vi "ScriptParser.vi"(0 "File Path Control":path, 1 "storage refnum (file) out":refnum<k20>, 2 "ResultaFileName":string, 3 "Array":string[](array[string]), 4 "I":dbl) -> ()   [LabVIEW 2014]
uses:
  <vilib>/Platform/storage/Storage.llb/usiSequenceRepresentation.ctl
  <vilib>/Platform/storage/lvStorage.llb/_queryPropPoly.vi
  <vilib>/Platform/storage/lvStorage.llb/_queryPropString.vi
  <vilib>/Platform/storage/lvStorage.llb/_queryGenericObjects.vi
  <vilib>/Platform/storage/lvStorage.llb/_loadAllDdt.vi
  <vilib>/Platform/storage/lvStorage.llb/xStorage/xStorageSupp/ErrorOut.vi
  <vilib>/Platform/storage/lvStorage.llb/_createOrGetByNameExplicitChildObject.vi
  <vilib>/Platform/storage/Storage.llb/__savePropString.vi
  <vilib>/Platform/storage/lvStorage.llb/__saveFloat64Channel.vi
  <vilib>/Platform/storage/lvStorage.llb/_openStorageWithRootAutoDetect.vi
  <vilib>/Platform/storage/Storage.llb/__savePropTime.vi
  <vilib>/Platform/storage/lvStorage.llb/xStorage/Read Data/Read Data.xnode
  <vilib>/Platform/storage/lvStorage.llb/xStorage/Write Data/Write Data.xnode
  <vilib>/Platform/storage/lvStorage.llb/xStorage/Open Data Storage/Open Data Storage.xnode
  <vilib>/Platform/storage/lvStorage.llb/xStorage/Set Properties/Set Properties.xnode
panel:
  out "Numeric":dbl
  out "storage refnums (channel)":refnum<k20>[](array[refnum])
  out "Default":bool
  # "DEBUG"
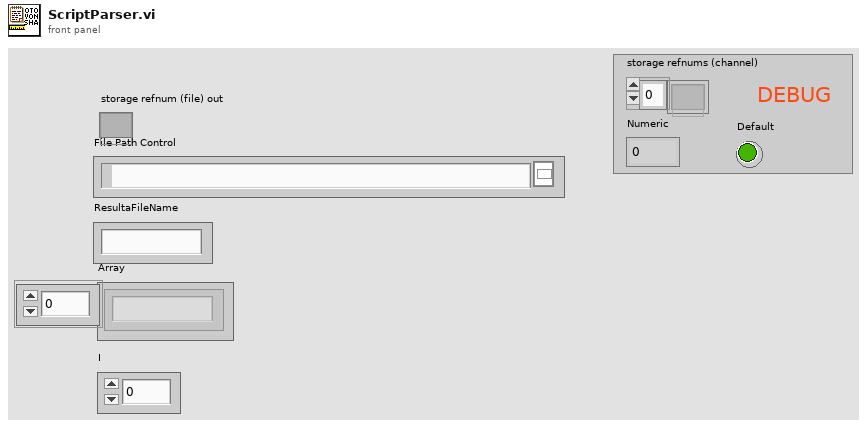
[diagram p1: front panel]
types:
  T1 = enum16{"UPDATE", "READ", "QUERY", "CREATE CHILD", "CREATE", "CONNECT", "DISCONNECT"}
  T2 = enum16{"Append values", "Replace values at index", "Replace all values"}
  T3 = typedef "usiSequenceRepresentation.ctl" = enum16{"explicit", "implicit"}
  T4 = enum16{"open", "open or create", "create or replace", "create", "open (read only)"}
  T5 = typedef "VBreakInitialCond.ctl" = cluster{"Range":dbl, "Ilim":dbl, "Level":dbl, "Channel":i32, "Timed Totalize":dbl}
  T6 = typedef "VBreakStopCondition.ctl" = cluster{"Count Min":dbl, "Count Max":dbl, "Vmax":dbl}
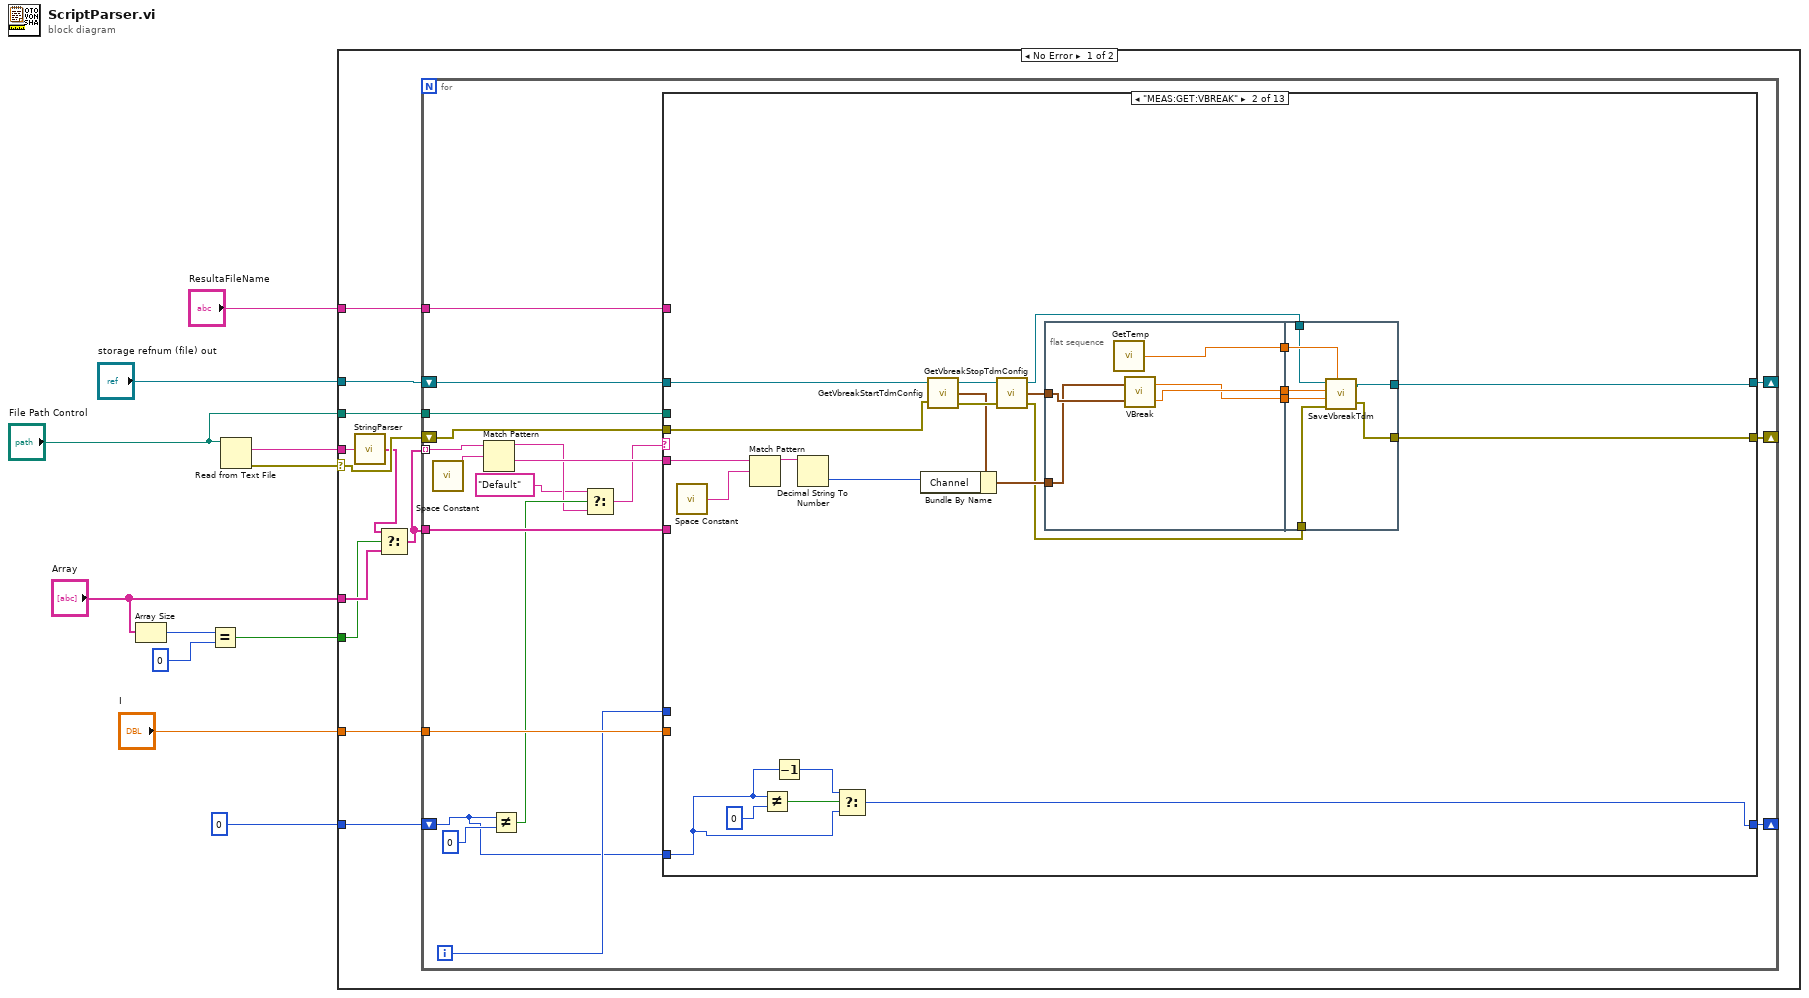
[diagram p0: block diagram]
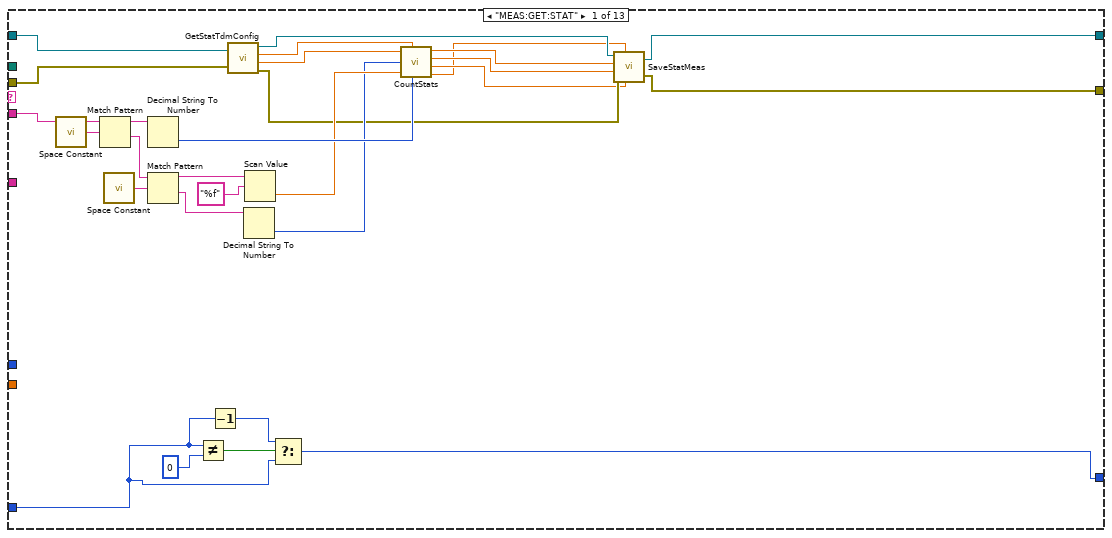
[diagram p2: hidden frame]
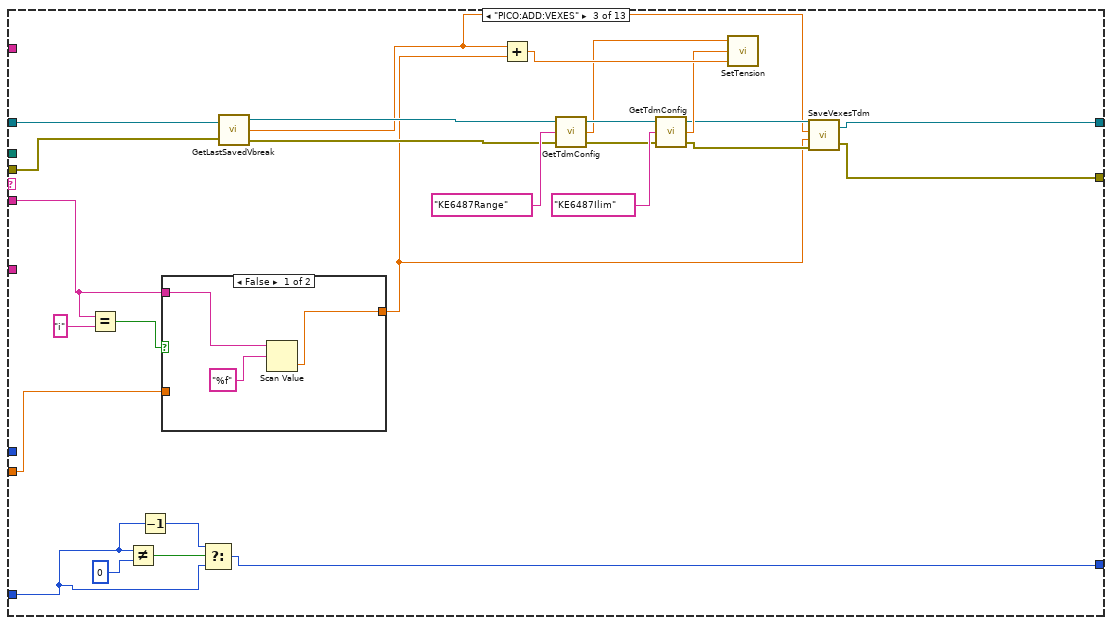
[diagram p3: hidden frame]
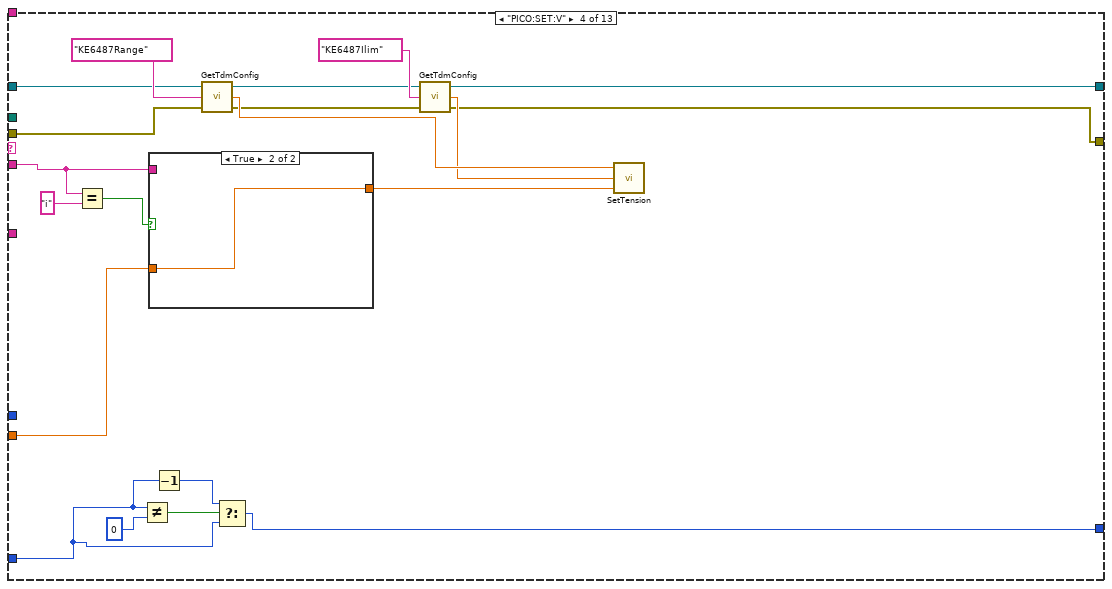
[diagram p5: hidden frame]
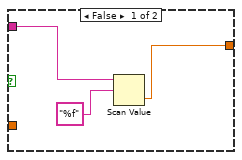
[diagram p6: hidden frame]
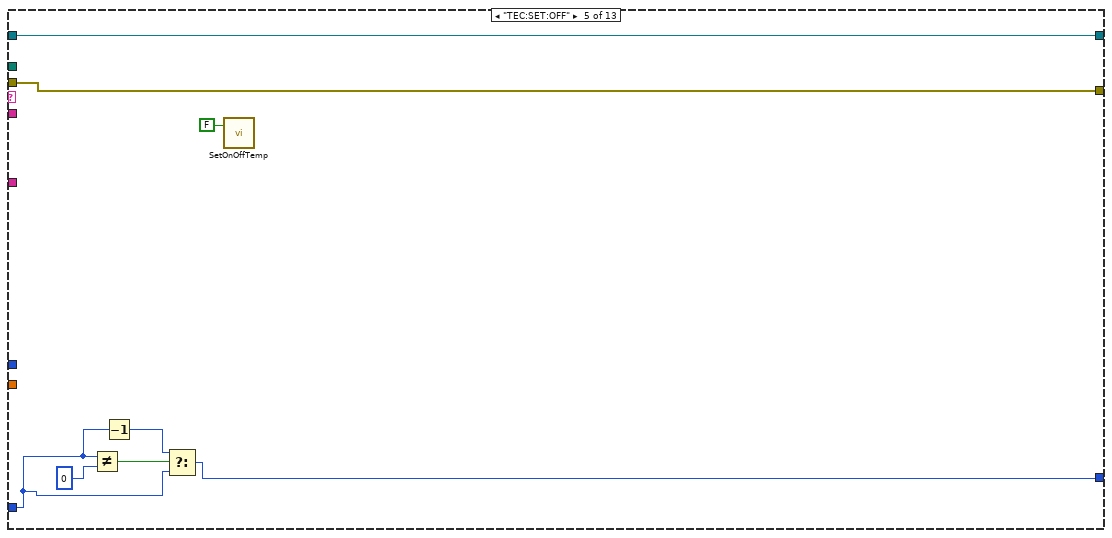
[diagram p7: hidden frame]
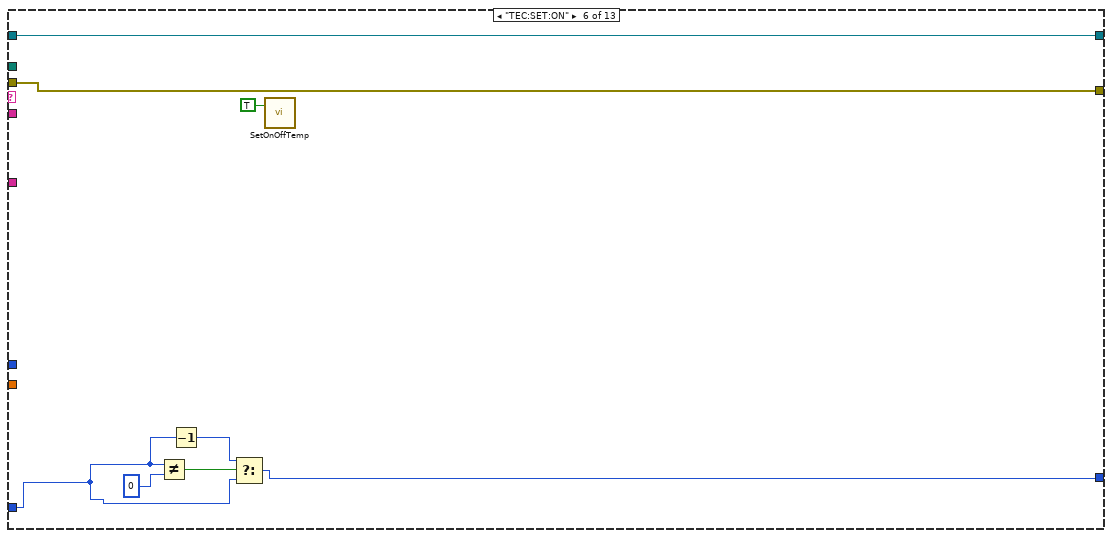
[diagram p8: hidden frame]
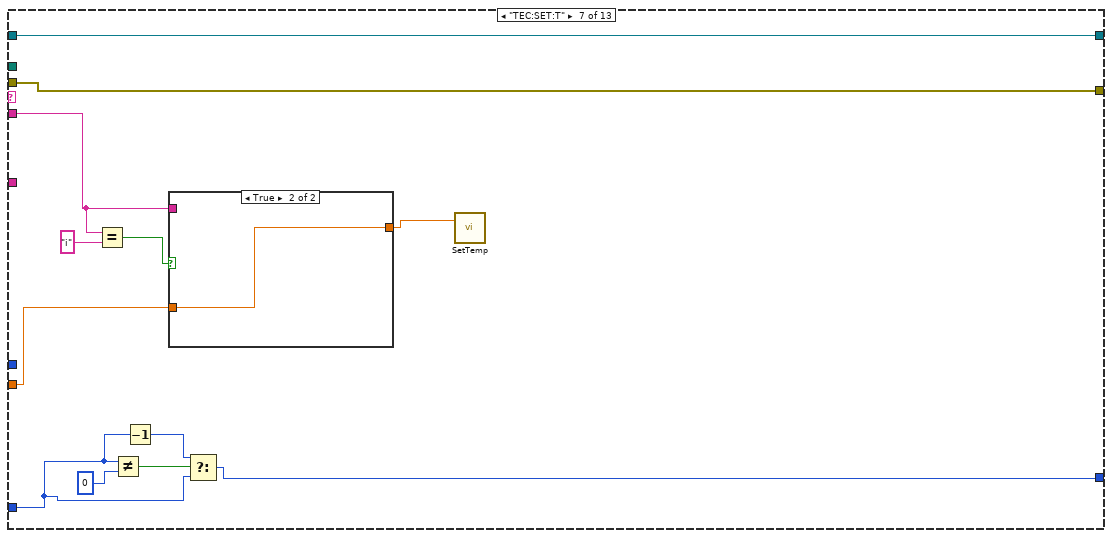
[diagram p9: hidden frame]
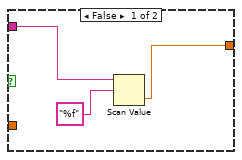
[diagram p10: hidden frame]
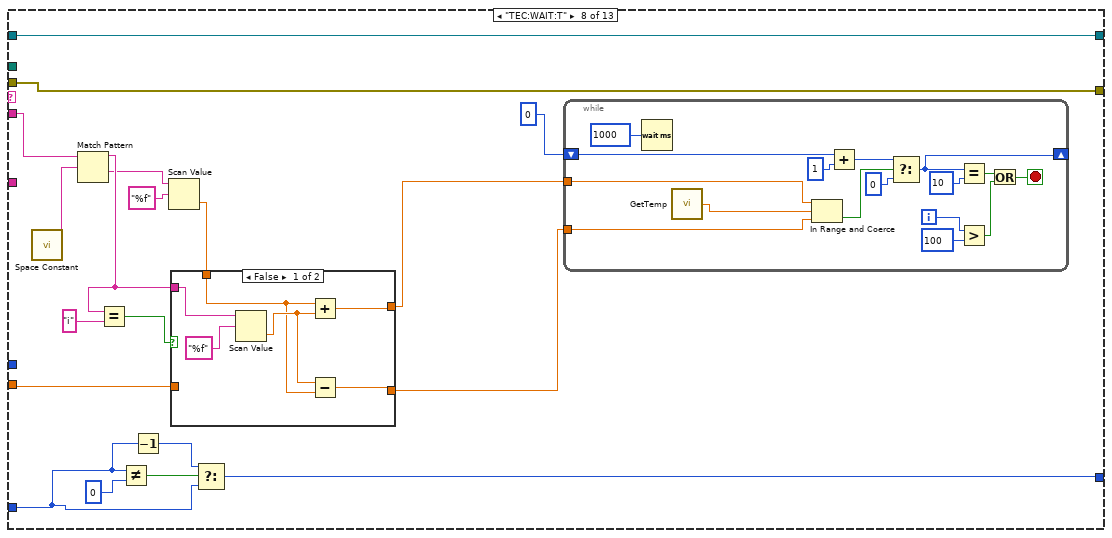
[diagram p11: hidden frame]
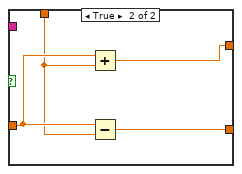
[diagram p12: hidden frame]
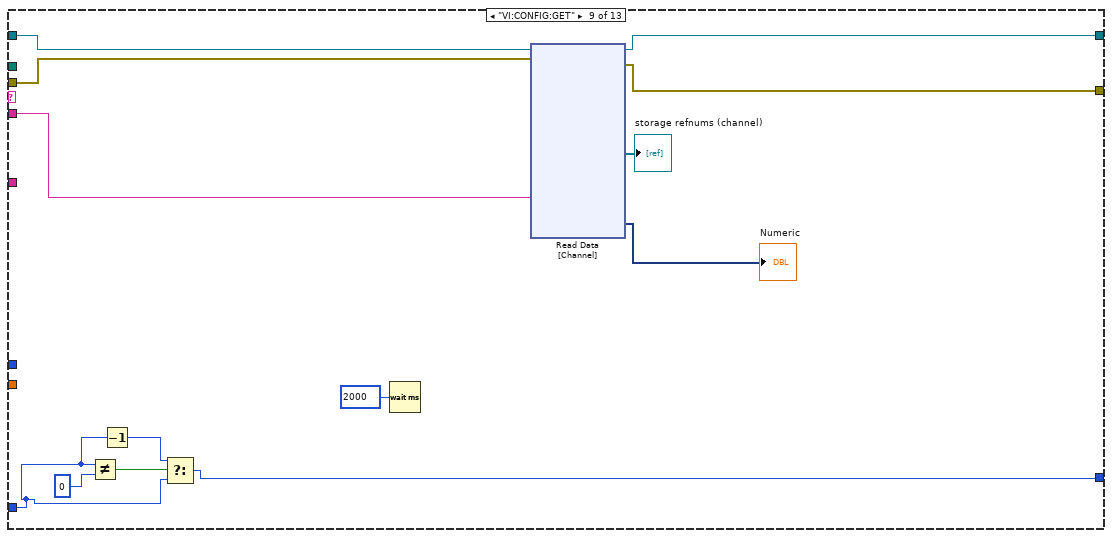
[diagram p13: hidden frame]
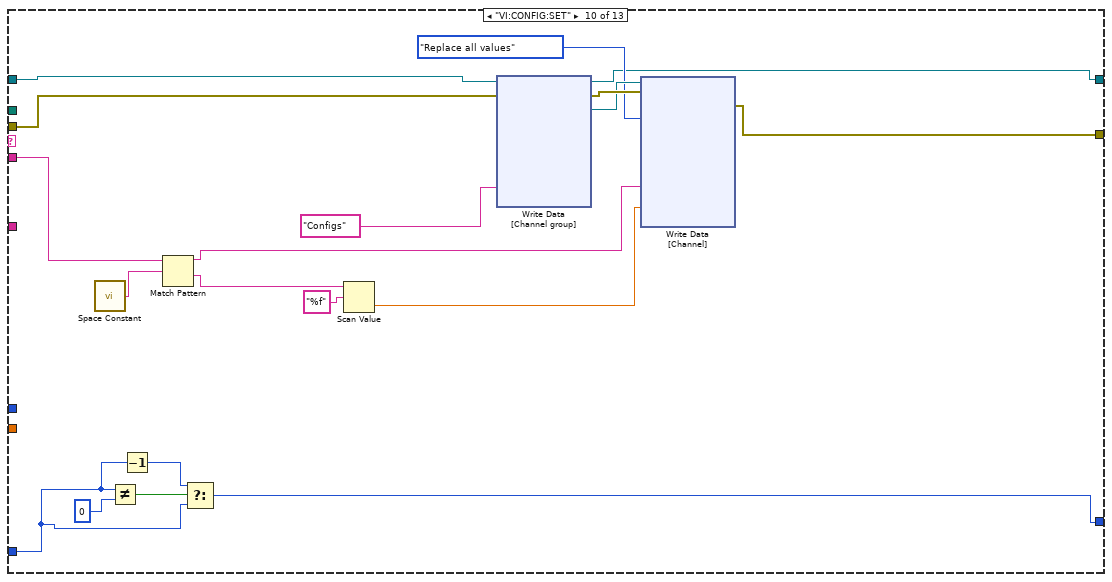
[diagram p14: hidden frame]
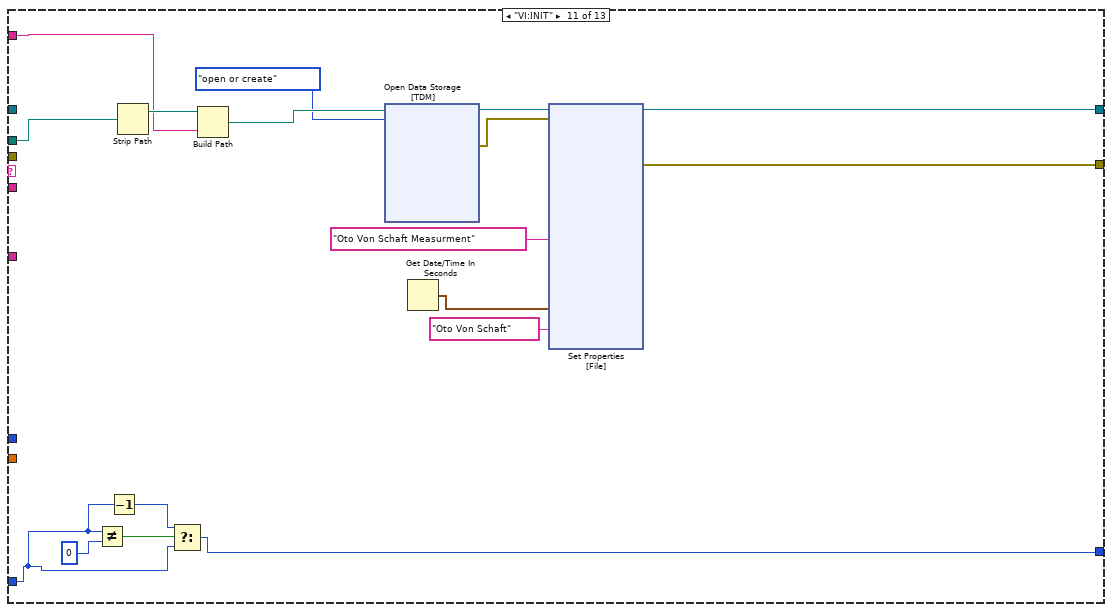
[diagram p15: hidden frame]
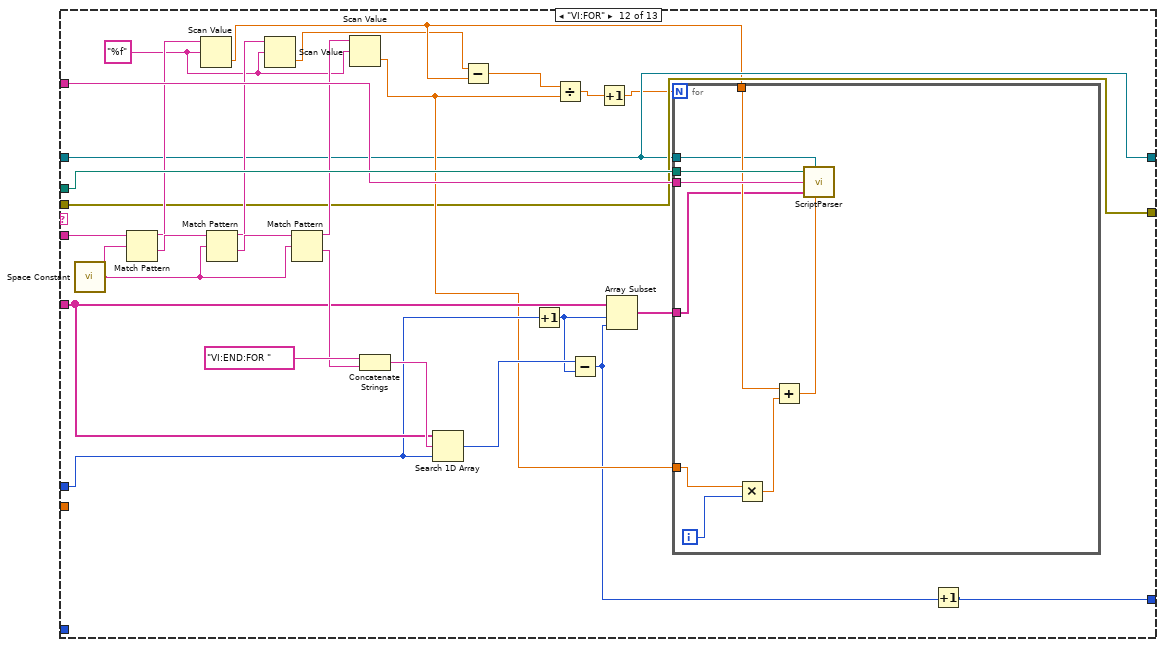
[diagram p16: hidden frame]
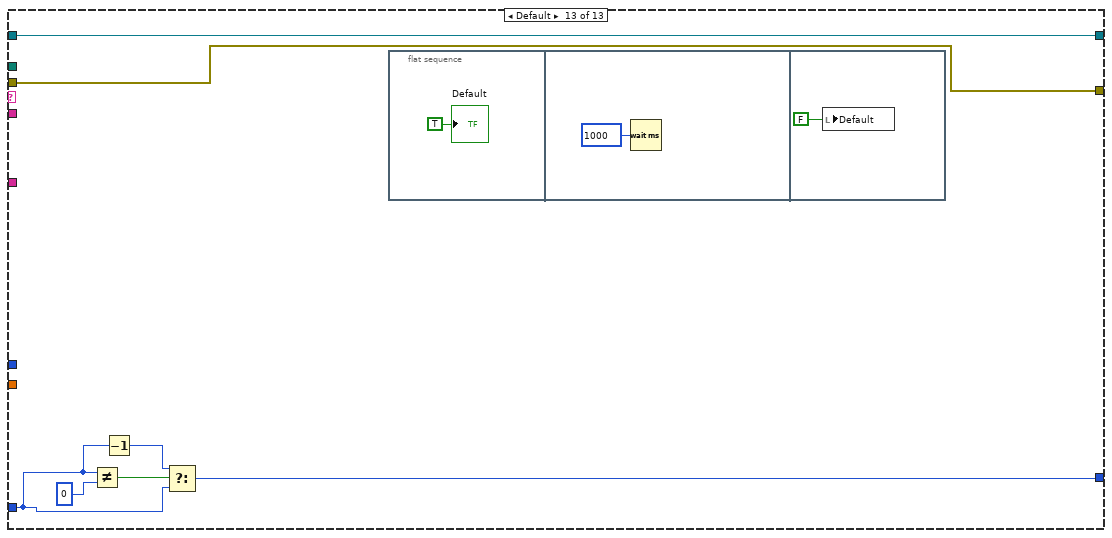
[diagram p17: hidden frame]
diagram:
  n1 = Array Size(array="Array") -> (size(s)=w4:i32)
  n2 = Equal?(x=w4, y=0) -> (x = y?=w2:bool)
  n3 = Read from Text File(file (use dialog)="File Path Control") -> (text=w6:string, error out=w11:errorcluster)  [unwired: 3 in, 2 out]
  n4 = case shown="No Error" w11 {
    selector: w11 -> [w20 _]
    tunnel: w6 -> [w18 _]
    tunnel: "File Path Control" -> [w22 _]
    tunnel: "ResultaFileName" -> [w21 _]
    tunnel: "I" -> [w19 _]
    tunnel: "storage refnum (file) out" -> [w17 _]
    tunnel: "Array" -> [w15 _]
    tunnel: w2 -> [w14 _]
    tunnel: 0 -> [w12 _]
    frame No Error {
      n5 = call "StringParser.vi"("String"=w18) -> ("array"=w16:string[])
      n6 = Select(t=w16, s=w14, f=w15) -> (s? t:f=w13:string[])
      n7 = for {
        tunnel: w13 -> [w40] mode=indexing
        tunnel: w22 -> [w35]
        tunnel: w21 -> [w38]
        shift-right: [w37] -> _
        shift-left: w17 -> [w34]
        shift-right: [w36] -> _
        shift-left: w20 -> [w33]
        tunnel: w19 -> [w32]
        tunnel: w13 -> [w31]
        shift-right: [w24] -> _
        shift-left: w12 -> [w23]
        i -> [w30]
        n8 = call <vilib>:"Space Constant.vi"() -> ("String"=w41:string)
        n9 = Match Pattern(string=w40, regular expression=w41) -> (before substring=w27:string, after substring=w39:string)  [unwired: 1 in, 2 out]
        n10 = Not Equal?(x=w23, y=0) -> (x != y?=w28:bool)
        n11 = Select(t="Default", s=w28, f=w27) -> (s? t:f=w25:string)
        n12 = case shown="\"MEAS:GET:VBREAK\"" w25 {
          tunnel: w39 -> [w66 w86 w112 w142 _ _ w181 w197 w248 w285 _ w397 _]
          tunnel: w35 -> [_ _ _ _ _ _ _ _ _ _ w333 w386 _]
          tunnel: w38 -> [_ _ _ _ _ _ _ _ _ _ w334 w384 _]
          tunnel: [w48 w71 w108 w146 w165 w173 w186 w207 w243 w274 w325 w376 w413] -> w37
          tunnel: [w47 w70 w107 w145 w164 w172 w185 w206 w242 w273 w324 w377 w412] -> w36
          tunnel: w34 -> [w69 w92 w130 w150 w165 w173 w186 w207 w244 w275 _ w376 w413]
          tunnel: w33 -> [w68 w91 w129 w149 w164 w172 w185 w206 w241 w272 _ w377 w412]
          tunnel: w32 -> [_ _ w111 w140 _ _ w182 w198 _ _ _ _ _]
          tunnel: w31 -> [_ _ _ _ _ _ _ _ _ _ _ w390 _]
          tunnel: w30 -> [_ _ _ _ _ _ _ _ _ _ _ w388 _]
          tunnel: [w42 w77 w117 w135 w159 w167 w175 w201 w236 w267 w319 w372 w407] -> w24
          tunnel: w23 -> [w43 w78 w118 w136 w160 w168 w176 w202 w237 w268 w320 _ w408]
          frame "MEAS:GET:STAT" {
            n13 = call <vilib>:"Space Constant.vi"() -> ("String"=w67:string)
            n14 = Match Pattern(string=w66, regular expression=w67) -> (before substring=w63:string, after substring=w60:string)  [unwired: 1 in, 2 out]
            n15 = call <vilib>:"Space Constant.vi"() -> ("String"=w61:string)
            n16 = Decimal String To Number(string=w63) -> (number=w62:i32)  [unwired: 2 in, 1 out]
            n17 = Match Pattern(string=w60, regular expression=w61) -> (before substring=w59:string, after substring=w57:string)  [unwired: 1 in, 2 out]
            n18 = Not Equal?(x=w43, y=0) -> (x != y?=w45:bool)
            n19 = Decrement(x=w43) -> (x-1=w44:i32)
            n20 = call "GetStatTdmConfig.vi"("storage refnum (file)"=w69, "error in"=w68) -> ("storage refnum (file) out"=w54:refnum<k20>, "Impedance"=w65:dbl, "Voltage Range"=w64:dbl, "error out"=w53:errorcluster)
            n21 = Decimal String To Number(string=w57) -> (number=w55:i32)  [unwired: 2 in, 1 out]
            n22 = Scan Value(string=w59, format string="%f") -> (value=w56:dbl)  [unwired: 1 in, 1 out]
            n23 = Select(t=w44, s=w45, f=w43) -> (s? t:f=w42:i32)
            n24 = call "CountStats.vi"("Voltage Range (5V)"=w64, "Impedance (1E+6 Ohm)"=w65, "Channel (Channel1)"=w55, "Totalize Timed (s)"=w56, "Points"=w62) -> ("Moyenne"=w52:dbl, "Ecart type"=w51:dbl, "Min"=w50:dbl, "Max"=w49:dbl)
            n25 = call "SaveStatMeas.vi"("Min"=w50, "Max"=w49, "error in"=w53, "Ecart Type"=w51, "Moyenne"=w52, "storage refnum (file)"=w54) -> ("error out"=w47:errorcluster, "storage refnum (file) 2"=w48:refnum<k20>)
          }
          frame "MEAS:GET:VBREAK" {
            n26 = call <vilib>:"Space Constant.vi"() -> ("String"=w87:string)
            n27 = Match Pattern(string=w86, regular expression=w87) -> (before substring=w85:string)  [unwired: 1 in, 3 out]
            n28 = Not Equal?(x=w78, y=0) -> (x != y?=w80:bool)
            n29 = Decrement(x=w78) -> (x-1=w79:i32)
            n30 = Decimal String To Number(string=w85) -> (number=w83:i32)  [unwired: 2 in, 1 out]
            n31 = Select(t=w79, s=w80, f=w78) -> (s? t:f=w77:i32)
            n32 = call "GetVbreakStartTdmConfig.vi"("storage refnum (file)"=w92, "error in"=w91) -> ("storage refnum (file) out"=w90:refnum<k20>, "output cluster"=w84:T5, "error out"=w89:errorcluster)
            n33 = Bundle By Name(cluster=w84, "Channel"=w83) -> (w82:T5)
            n34 = call "GetVbreakStopTdmConfig.vi"("storage refnum (file)"=w90, "error in"=w89) -> ("storage refnum (file) out"=w73:refnum<k20>, "output cluster"=w88:T6, "error out"=w72:errorcluster)
            n35 = flat-sequence {
              tunnel: w88 -> [w97]
              tunnel: w82 -> [w93]
              tunnel: [w96] -> w76
              tunnel: [w95] -> w75
              tunnel: [w94] -> w74
              tunnel: w76 -> [w103]
              tunnel: w75 -> [w102]
              tunnel: w74 -> [w104]
              tunnel: w73 -> [w100]
              tunnel: w72 -> [w101]
              tunnel: [w99] -> w71
              tunnel: [w98] -> w70
              frame #0 {
                n36 = call "GetTemp.vi"() -> ("result"=w94:dbl)
                n37 = call "VBreak.vi"("Condition d'arret"=w97, "Condition Initial"=w93) -> ("VBreak"=w96:dbl, "Count"=w95:dbl)
              }
              frame #1 {
                n38 = call "SaveVbreakTdm.vi"("storage refnum (file)"=w100, "Vbreak"=w103, "Count"=w102, "error in"=w101, "Temp"=w104) -> ("storage refnum (file) 2"=w99:refnum<k20>, "error out"=w98:errorcluster)
              }
            }
          }
          frame "PICO:ADD:VEXES" {
            n39 = Equal?(x=w112, y="i") -> (x = y?=w113:bool)
            n40 = Not Equal?(x=w118, y=0) -> (x != y?=w120:bool)
            n41 = Decrement(x=w118) -> (x-1=w119:i32)
            n42 = case shown="False" w113 {
              tunnel: w112 -> [w132 _]
              tunnel: [w131 w134] -> w105
              tunnel: w111 -> [_ w134]
              frame False {
                n43 = Scan Value(string=w132, format string="%f") -> (value=w131:dbl)  [unwired: 1 in, 1 out]
              }
              frame True {
              }
            }
            n44 = Select(t=w119, s=w120, f=w118) -> (s? t:f=w117:i32)
            n45 = call "GetLastSavedVbreak.vi"("storage refnum (file)"=w130, "error in"=w129) -> ("storage refnum (file) out"=w116:refnum<k20>, "VBreak"=w106:dbl, "error out"=w115:errorcluster)
            n46 = Add(x=w106, y=w105) -> (x+y=w124:dbl)
            n47 = call "GetTdmConfig.vi"("error in 2"=w115, "String"="KE6487Range", "storage refnum (file)"=w116) -> ("error in"=w125:errorcluster, "Numeric"=w123:dbl, "storage refnum (file) out"=w126:refnum<k20>)
            n48 = call "GetTdmConfig.vi"("error in 2"=w125, "String"="KE6487Ilim", "storage refnum (file)"=w126) -> ("error in"=w109:errorcluster, "Numeric"=w122:dbl, "storage refnum (file) out"=w110:refnum<k20>)
            n49 = call "SetTension.vi"("level"=w124, "compliance limit"=w122, "range"=w123) -> ()
            n50 = call "SaveVexesTdm.vi"("error in"=w109, "VExes"=w105, "Vbreak"=w106, "storage refnum (file)"=w110) -> ("error out"=w107:errorcluster, "storage refnum (file) 3"=w108:refnum<k20>)
          }
          frame "PICO:SET:V" {
            n51 = Equal?(x=w142, y="i") -> (x = y?=w143:bool)
            n52 = Not Equal?(x=w136, y=0) -> (x != y?=w138:bool)
            n53 = case shown="True" w143 {
              tunnel: w142 -> [w156 _]
              tunnel: [w155 w158] -> w141
              tunnel: w140 -> [_ w158]
              frame False {
                n54 = Scan Value(string=w156, format string="%f") -> (value=w155:dbl)  [unwired: 1 in, 1 out]
              }
              frame True {
              }
            }
            n55 = Decrement(x=w136) -> (x-1=w137:i32)
            n56 = call "GetTdmConfig.vi"("error in 2"=w149, "String"="KE6487Range", "storage refnum (file)"=w150) -> ("error in"=w147:errorcluster, "Numeric"=w154:dbl, "storage refnum (file) out"=w148:refnum<k20>)
            n57 = Select(t=w137, s=w138, f=w136) -> (s? t:f=w135:i32)
            n58 = call "GetTdmConfig.vi"("error in 2"=w147, "String"="KE6487Ilim", "storage refnum (file)"=w148) -> ("error in"=w145:errorcluster, "Numeric"=w153:dbl, "storage refnum (file) out"=w146:refnum<k20>)
            n59 = call "SetTension.vi"("level"=w141, "compliance limit"=w153, "range"=w154) -> ()
          }
          frame "TEC:SET:OFF" {
            n60 = Not Equal?(x=w160, y=0) -> (x != y?=w162:bool)
            n61 = Decrement(x=w160) -> (x-1=w161:i32)
            n62 = Select(t=w161, s=w162, f=w160) -> (s? t:f=w159:i32)
            n63 = call "SetOnOffTemp.vi"("Boolean"=FALSE) -> ()  [unwired: 1 in, 1 out]
          }
          frame "TEC:SET:ON" {
            n64 = Not Equal?(x=w168, y=0) -> (x != y?=w170:bool)
            n65 = Decrement(x=w168) -> (x-1=w169:i32)
            n66 = Select(t=w169, s=w170, f=w168) -> (s? t:f=w167:i32)
            n67 = call "SetOnOffTemp.vi"("Boolean"=TRUE) -> ()  [unwired: 1 in, 1 out]
          }
          frame "TEC:SET:T" {
            n68 = Equal?(x=w181, y="i") -> (x = y?=w183:bool)
            n69 = Not Equal?(x=w176, y=0) -> (x != y?=w178:bool)
            n70 = Decrement(x=w176) -> (x-1=w177:i32)
            n71 = case shown="True" w183 {
              tunnel: w181 -> [w188 _]
              tunnel: [w187 w190] -> w180
              tunnel: w182 -> [_ w190]
              frame False {
                n72 = Scan Value(string=w188, format string="%f") -> (value=w187:dbl)  [unwired: 1 in, 1 out]
              }
              frame True {
              }
            }
            n73 = Select(t=w177, s=w178, f=w176) -> (s? t:f=w175:i32)
            n74 = call "SetTemp.vi"("Numeric Control"=w180) -> ()  [unwired: 1 in, 1 out]
          }
          frame "TEC:WAIT:T" {
            n75 = call <vilib>:"Space Constant.vi"() -> ("String"=w209:string)
            n76 = Match Pattern(string=w197, regular expression=w209) -> (before substring=w196:string, after substring=w194:string)  [unwired: 1 in, 2 out]
            n77 = Equal?(x=w196, y="i") -> (x = y?=w199:bool)
            n78 = Not Equal?(x=w202, y=0) -> (x != y?=w204:bool)
            n79 = Decrement(x=w202) -> (x-1=w203:i32)
            n80 = Scan Value(string=w194, format string="%f") -> (value=w193:dbl)  [unwired: 1 in, 1 out]
            n81 = case shown="False" w199 {
              tunnel: w196 -> [w214 _]
              tunnel: [w210 w217] -> w192
              tunnel: w198 -> [_ w219]
              tunnel: w193 -> [w212 w218]
              tunnel: [w211 w216] -> w191
              frame False {
                n82 = Scan Value(string=w214, format string="%f") -> (value=w213:dbl)  [unwired: 1 in, 1 out]
                n83 = Add(x=w212, y=w213) -> (x+y=w210:dbl)
                n84 = Subtract(x=w213, y=w212) -> (x-y=w211:dbl)
              }
              frame True {
                n85 = Add(x=w219, y=w218) -> (x+y=w217:dbl)
                n86 = Subtract(x=w219, y=w218) -> (x-y=w216:dbl)
              }
            }
            n87 = Select(t=w203, s=w204, f=w202) -> (s? t:f=w201:i32)
            n88 = while {
              tunnel: w192 -> [w234]
              tunnel: w191 -> [w235]
              shift-right: [w228] -> _
              shift-left: 0 -> [w231]
              i -> [w224]
              stop <- w225 stop-if-true
              n89 = Wait (ms)(milliseconds to wait=u32 1000) -> ()  [unwired: 1 out]
              n90 = call "GetTemp.vi"() -> ("result"=w220:dbl)
              n91 = In Range and Coerce(upper limit=w234, x=w220, lower limit=w235) -> (In Range?=w233:bool)  [unwired: 1 out]
              n92 = Add(x=w231, y=1) -> (x+y=w229:i32)
              n93 = Select(t=w229, s=w233, f=0) -> (s? t:f=w228:i32)
              n94 = Equal?(x=w228, y=10) -> (x = y?=w226:bool)
              n95 = Greater?(x=w224, y=100) -> (0:w222:bool)
              n96 = Or(x=w226, y=w222) -> (x .or. y?=w225:bool)
            }
          }
          frame "VI:CONFIG:GET" {
            n97 = Not Equal?(x=w237, y=0) -> (x != y?=w239:bool)
            n98 = Decrement(x=w237) -> (x-1=w238:i32)
            n99 = Select(t=w238, s=w239, f=w237) -> (s? t:f=w236:i32)
            n100 = Wait (ms)(milliseconds to wait=u32 2000) -> ()  [unwired: 1 out]
            n101 = xnode "Read Data\n[Channel]"("Name"=w248, "storage refnum (file)"=w244, "error in"=w241) -> ("storage refnums (channel)"=→"storage refnums (channel)":refnum<k20>[], "Signal"=→"Numeric":dynamicdata, "storage refnum (file) out"=w243:refnum<k20>, "error out"=w242:errorcluster)  [unwired: 3 in]
          }
          frame "VI:CONFIG:SET" {
            n102 = call <vilib>:"Space Constant.vi"() -> ("String"=w284:string)
            n103 = Not Equal?(x=w268, y=0) -> (x != y?=w270:bool)
            n104 = Decrement(x=w268) -> (x-1=w269:i32)
            n105 = Match Pattern(string=w285, regular expression=w284) -> (before substring=w283:string, after substring=w282:string)  [unwired: 1 in, 2 out]
            n106 = Select(t=w269, s=w270, f=w268) -> (s? t:f=w267:i32)
            n107 = Scan Value(string=w282, format string="%f") -> (value=w280:dbl)  [unwired: 1 in, 1 out]
            n108 = xnode "Write Data\n[Channel group]"("Name"="Configs", "storage refnum (file)"=w275, "error in"=w272) -> ("storage refnum (file) out"=w274:refnum<k20>, "error out"=w279:errorcluster, "storage refnum (channel group)"=w277:refnum<k20>)
            n109 = xnode "Write Data\n[Channel]"("Name"=w283, "Signal"=w280, "storage refnum (channel group)"=w277, "error in"=w279, "append / replace (append data values)"=T2."Replace all values") -> ("error out"=w273:errorcluster)  [unwired: 1 in, 2 out]
          }
          frame "VI:INIT" {
            n110 = Not Equal?(x=w320, y=0) -> (x != y?=w322:bool)
            n111 = Decrement(x=w320) -> (x-1=w321:i32)
            n112 = Strip Path(path=w333) -> (stripped path=w335:path)  [unwired: 1 out]
            n113 = Select(t=w321, s=w322, f=w320) -> (s? t:f=w319:i32)
            n114 = Build Path(base path=w335, name or relative path=w334) -> (appended path=w332:path)
            n115 = xnode "Open Data Storage\n[TDM]"("file path"=w332, "function (open:0)"=T4."open or create") -> ("storage refnum (file)"=w330:refnum<k20>, "error out"=w329:errorcluster)  [unwired: 3 in, 1 out]
            n116 = Get Date/Time In Seconds() -> (seconds since 1Jan1904=w327:timestamp)
            n117 = xnode "Set Properties\n[File]"("Name"="Oto Von Schaft Measurment", "Time stamp"=w327, "Author"="Oto Von Schaft", "storage refnum (file)"=w330, "error in"=w329) -> ("storage refnum (file) out"=w325:refnum<k20>, "error out"=w324:errorcluster)  [unwired: 2 in]
          }
          frame "VI:FOR" {
            w380 = "%f" ("format string")
            n118 = call <vilib>:"Space Constant.vi"() -> ("String"=w394:string)
            n119 = Match Pattern(string=w397, regular expression=w394) -> (before substring=w383:string, after substring=w396:string)  [unwired: 1 in, 2 out]
            n120 = Scan Value(string=w383, format string=w380) -> (value=w375:dbl)  [unwired: 1 in, 1 out]
            n121 = Match Pattern(string=w396, regular expression=w394) -> (before substring=w382:string, after substring=w395:string)  [unwired: 1 in, 2 out]
            n122 = Scan Value(string=w382, format string=w380) -> (value=w374:dbl)  [unwired: 1 in, 1 out]
            n123 = Match Pattern(string=w395, regular expression=w394) -> (before substring=w381:string, after substring=w392:string)  [unwired: 1 in, 2 out]
            n124 = Scan Value(string=w381, format string=w380) -> (value=w378:dbl)  [unwired: 1 in, 1 out]
            n125 = Concatenate Strings("VI:END:FOR " ("string"), w392) -> (w391:string)
            n126 = Search 1D Array(1D array=w390, element=w391, start index (0)=w388) -> (index of element=w389:i32)
            n127 = Subtract(x=w374, y=w375) -> (x-y=w379:dbl)
            n128 = Increment(x=w388) -> (x+1=w387:i32)
            n129 = Divide(x=w379, y=w378) -> (x/y=w371:dbl)
            n130 = Subtract(x=w389, y=w387) -> (x-y=w373:i32)
            n131 = Increment(x=w371) -> (x+1=w370:dbl)
            n132 = Array Subset(array=w390, index=w387, length=w373) -> (w385:string[])
            n133 = for {
              N: w370 -> [_]
              tunnel: w386 -> [w406]
              tunnel: w376 -> [w400]
              tunnel: w385 -> [w398]
              tunnel: w384 -> [w405]
              tunnel: w375 -> [w404]
              tunnel: w378 -> [w403]
              i -> [w399]
              n134 = Multiply(x=w403, y=w399) -> (x*y=w402:dbl)
              n135 = Add(x=w404, y=w402) -> (x+y=w401:dbl)
              n136 = call "ScriptParser.vi"("File Path Control"=w406, "storage refnum (file) out"=w400, "ResultaFileName"=w405, "Array"=w398, "I"=w401) -> ()  [unwired: 1 in]
            }
            n137 = Increment(x=w373) -> (x+1=w372:i32)
          }
          frame Default {
            n138 = Not Equal?(x=w408, y=0) -> (x != y?=w410:bool)
            n139 = Decrement(x=w408) -> (x-1=w409:i32)
            n140 = Select(t=w409, s=w410, f=w408) -> (s? t:f=w407:i32)
            n141 = flat-sequence {
              frame #0 {
                "Default" <- TRUE ("PicoSetV")
              }
              frame #1 {
                n142 = Wait (ms)(milliseconds to wait=u32 1000) -> ()  [unwired: 1 out]
              }
              frame #2 {
                n143 = local write "Default"(FALSE ("PicoSetV")) -> ()
              }
            }
          }
        }
      }
    }
    frame Error {
    }
  }
